vi "GetGpsData.vi"() -> (6 "latDeg":dbl format="%_6g", 7 "LonDeg":dbl format="%_6g", 8 "Sat":i32)   [LabVIEW 2017]
uses:
  <vilib>/Instr/_visa.llb/VISA Configure Serial Port (Instr).vi
  GlobalVarStop.vi
panel:
  out "Check":string
  out "error out":errorcluster
  out "Longitude (W)":dbl format="%#_8g"
  out "Latitude (N)":dbl format="%#_8g"
  out "Longitude [deg]":string
  out "Latitude [deg]":string
  in  "time zone":i32
  out "Time":string
  out "Mode":string
  out "Date [ddmmyy]":string
  out "Course over ground [degrees]":string
  out "Status":string
  out "Speed over ground [knots]":string
  out "E/W":string
  out "Longitude":string
  out "N/S":string
  out "Latitude":string
  out "UTC Time":string
  out "NMEA sentences":string
  # "GPS demo"
  # "[hhmmss.sss]"
  # "Floating Point Values"
  # "A = vAlid data\nV = inValid data"
  # "[ddmm.mmmm]"
  # "[dddmm.mmmm]"
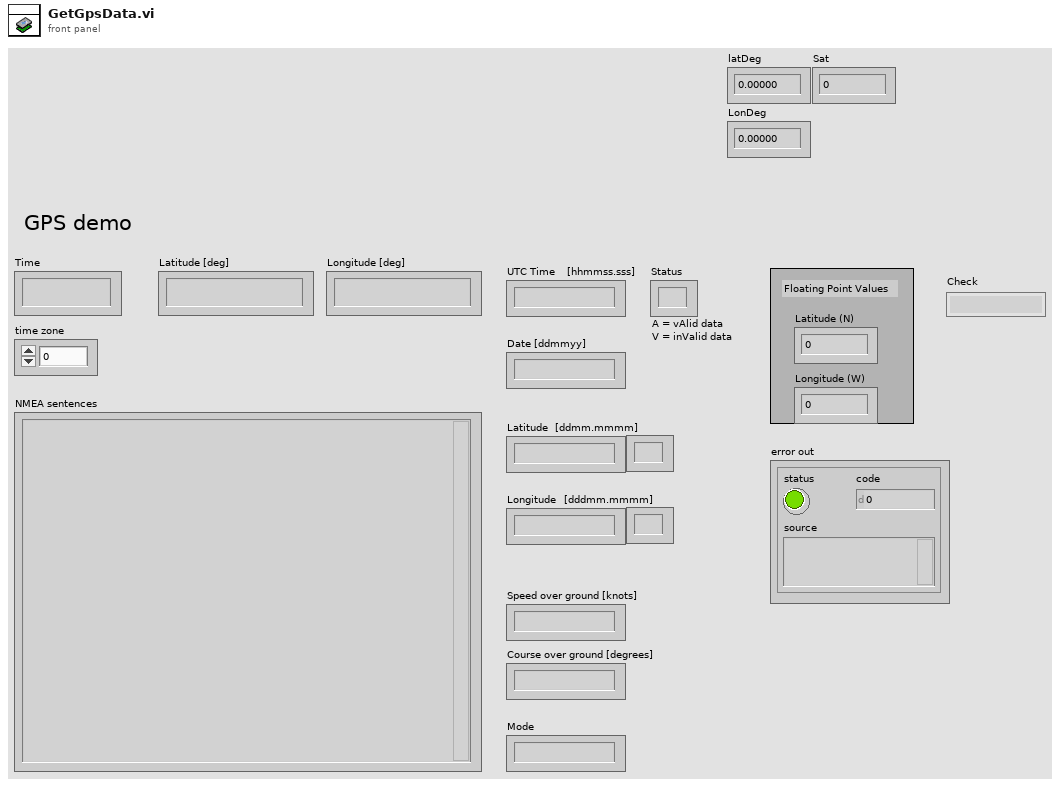
[diagram p1: front panel]
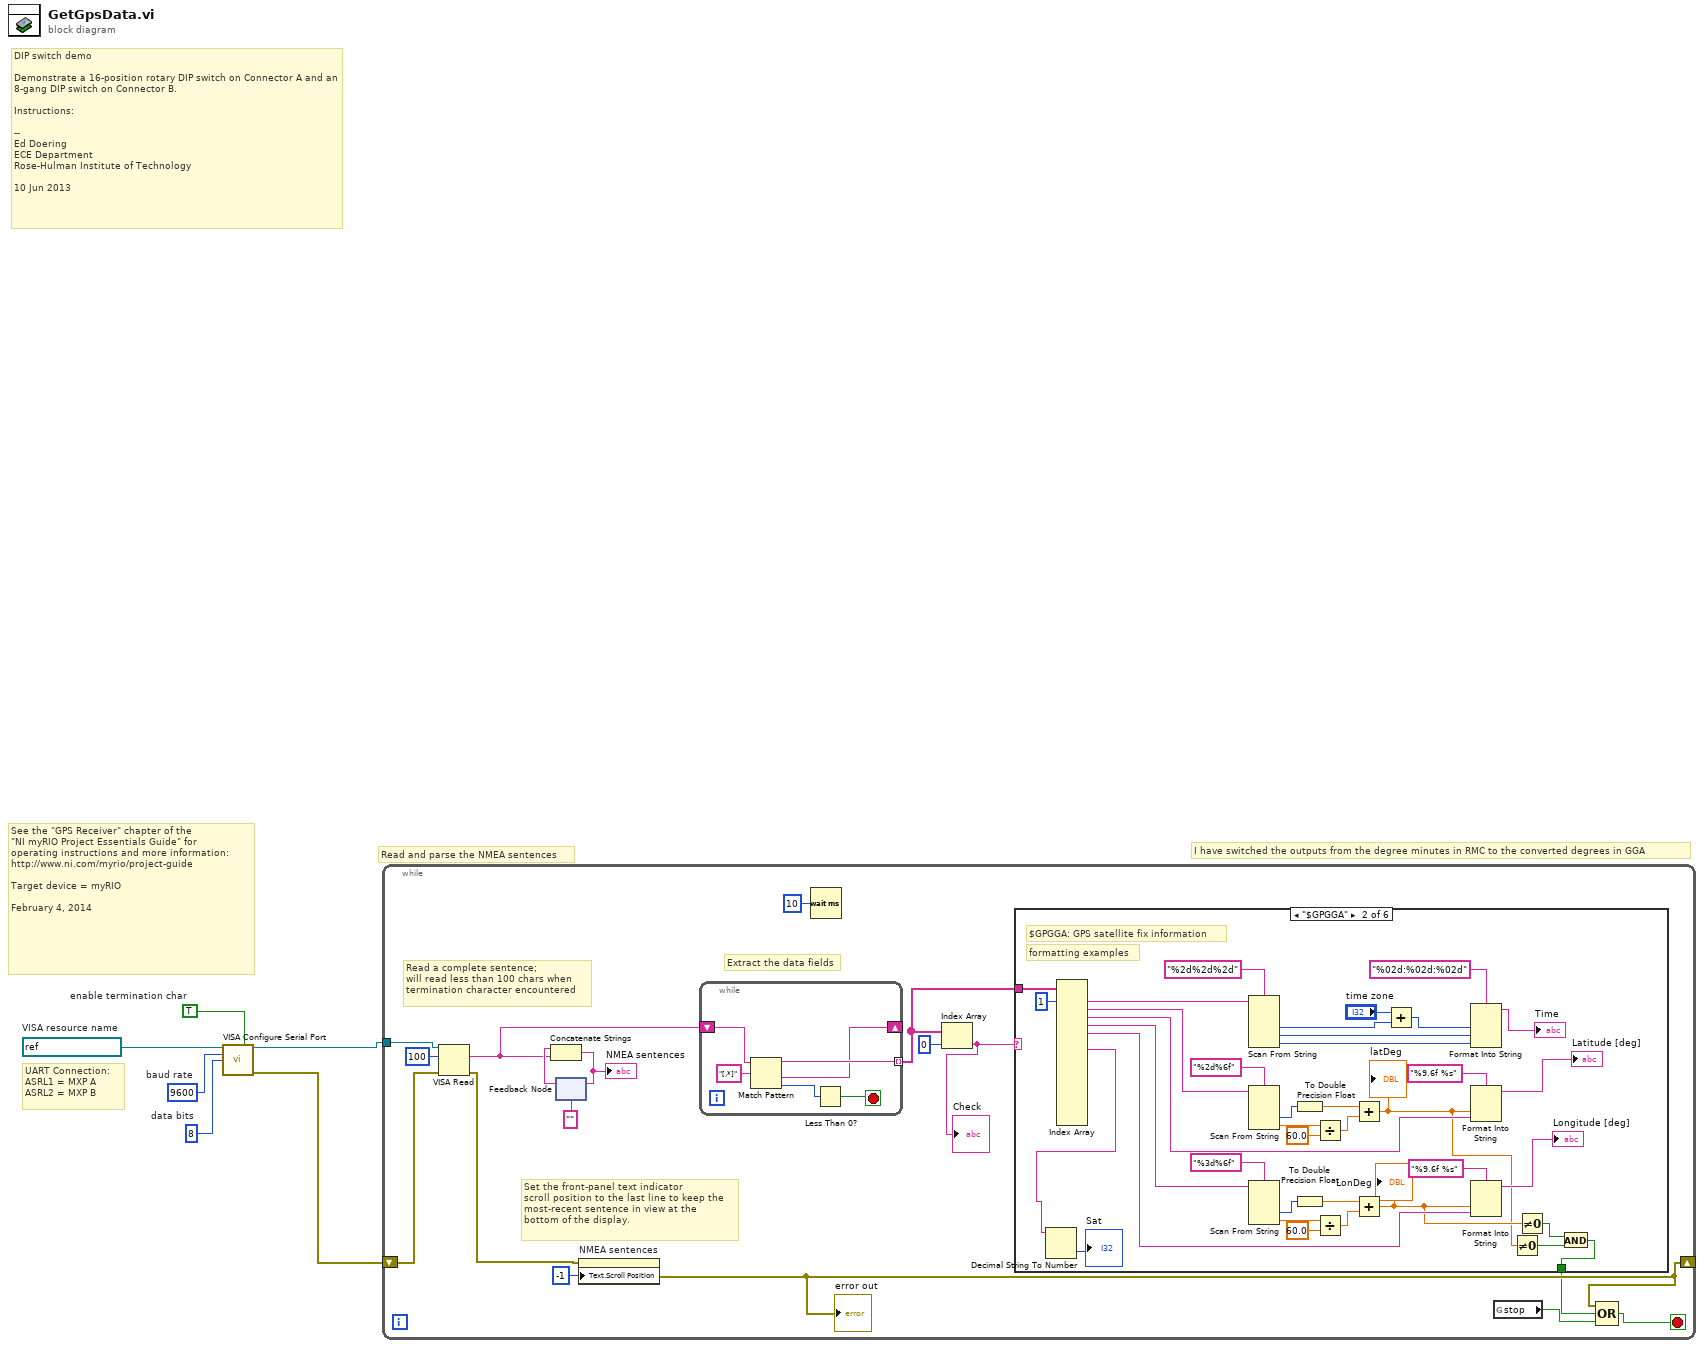
[diagram p0: block diagram]
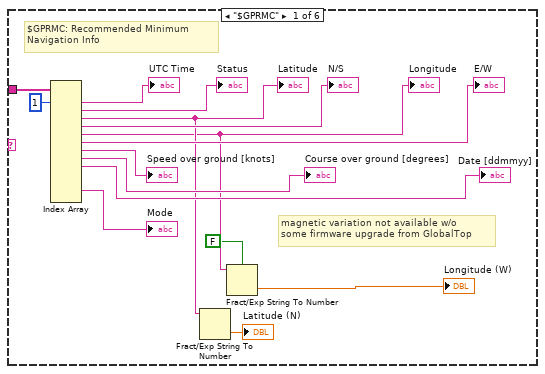
[diagram p2: hidden frame]
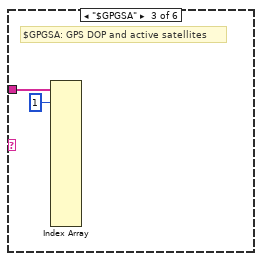
[diagram p3: hidden frame]
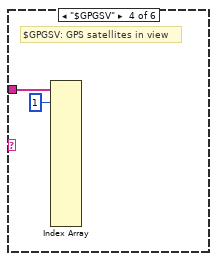
[diagram p4: hidden frame]
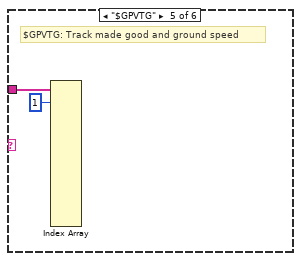
[diagram p5: hidden frame]
diagram:
  w2 = TRUE  # enable termination char
  w3 = u16 8  # data bits
  w4 = u32 9600  # baud rate
  w6 = refnum<visa-resource-name> "ASRL2::INSTR"  # VISA resource name
  # "I have switched the outputs from the degree minutes in RMC to the converted degrees in GGA"
  # "Read and parse the NMEA sentences"
  # "See the \"GPS Receiver\" chapter of the\n\"NI myRIO Project Essentials Guide\" for\noperating instructions and more information: \nhttp://www.ni.com/myrio/project-guide\n\nTarget device = myRIO\n\nFebruary 4, 2014"
  # "UART Connection:\nASRL1 = MXP A \nASRL2 = MXP B"
  # "DIP switch demo\n\nDemonstrate a 16-position rotary DIP switch on Connector A and an 8-gang DIP switch on Connector B.\n\nInstructions:\n\n-- \nEd Doering\nECE Department\nRose-Hulman Institute of Technology\n\n10 Jun 2013"
  n1 = call-poly "VISA Configure Serial Port"("VISA resource name"=w6, "Enable Termination\nChar (T)"=w2, "baud rate (9600)"=w4, "data bits (8)"=w3) -> ("VISA resource name out"=w5:refnum<visa-resource-name>, "error out"=w1:errorcluster)  [unwired: 10 in]
  n2 = while {
    tunnel: w5 -> [w23]
    shift-right: [w22] -> _
    shift-left: w1 -> [w21]
    stop <- w10 stop-if-true
    # "Set the front-panel text indicator\nscroll position to the last line to keep the\nmost-recent sentence in view at the\nbottom of the display."
    # "Extract the data fields"
    # "Read a complete sentence;\nwill read less than 100 chars when\ntermination character encountered"
    n3 = VISA Read(VISA resource name=w23, byte count=u32 100, error in (no error)=w21) -> (read buffer=w16:string, error out=w12:errorcluster)  [unwired: 2 out]
    n4 = feedback #1("") -> (w18:string)
    n5 = Concatenate Strings "Concatenate Strings"(w18, w16) -> (w20:string)
    "NMEA sentences" <- w20
    n6 = feedback-in #1(w20) -> ()
    n7 = property on="NMEA sentences" class="Str"(error in=w12, "Text.Scroll Position"=-1) -> (error out=w22:errorcluster)  [unwired: 1 in, 1 out]
    "error out" <- w22
    n8 = while {
      tunnel: [w86] -> w15 mode=indexing
      shift-right: [w85] -> _
      shift-left: w16 -> [w87]
      stop <- w84 stop-if-true
      n9 = Match Pattern(string=w87, regular expression="[,*]") -> (before substring=w86:string, after substring=w85:string, offset past match=w83:i32)  [unwired: 1 in, 1 out]
      n10 = Less Than 0?(x=w83) -> (x < 0?=w84:bool)
    }
    n11 = Wait (ms)(milliseconds to wait=u32 10) -> ()  [unwired: 1 out]
    n12 = Index Array "Index Array"(array=w15, index=0) -> (element=w7:string)
    "Check" <- w7
    n13 = case shown="\"$GPGGA\"" w7 {
      tunnel: w15 -> [w38 w76 w78 w80 w82 _]
      tunnel: [_ w41 _ _ _ _] -> w11
      frame "$GPRMC" {
        # "magnetic variation not available w/o\nsome firmware upgrade from GlobalTop"
        # "$GPRMC: Recommended Minimum\nNavigation Info"
        n14 = Index Array "Index Array"(array=w38, index #1=1 ("index")) -> (element #1=→"UTC Time":string, element #2=→"Status":string, element #3=w28:string, element #4=→"N/S":string, element #5=w27:string, element #6=→"E/W":string, element #7=→"Speed over ground [knots]":string, element #8=→"Course over ground [degrees]":string, element #9=→"Date [ddmmyy]":string, element #12=→"Mode":string)  [unwired: 12 in, 3 out]
        "Latitude" <- w28
        "Longitude" <- w27
        n15 = Fract/Exp String To Number(string=w28) -> (number=→"Latitude (N)":dbl)  [unwired: 3 in, 1 out]
        n16 = Fract/Exp String To Number(use system decimal point (T)=FALSE, string=w27) -> (number=→"Longitude (W)":dbl)  [unwired: 2 in, 1 out]
      }
      frame "$GPGGA" {
        # "formatting examples"
        # "$GPGGA: GPS satellite fix information"
        n17 = Index Array "Index Array"(array=w76, index #1=1 ("index")) -> (element #1=w73:string, element #2=w64:string, element #3=w57:string, element #4=w47:string, element #5=w46:string, element #7=w45:string)  [unwired: 15 in, 10 out]
        n18 = Decimal String To Number(string=w45) -> (number=→"Sat":i32)  [unwired: 2 in, 1 out]
        n19 = Scan From String "Scan From String"(format string="%2d%2d%2d", input string=w73) -> (output 1=w66:i32, output 2=w69:i32, output 3=w71:i32)  [unwired: 5 in, 3 out]
        n20 = Scan From String(format string="%2d%6f", input string=w64) -> (output 1=w61:i32, output 2=w63:dbl)  [unwired: 4 in, 3 out]
        n21 = Scan From String(format string="%3d%6f", input string=w47) -> (output 1=w51:i32, output 2=w49:dbl)  [unwired: 4 in, 3 out]
        n22 = To Double Precision Float(number=w61) -> (double precision float=w59:dbl)
        n23 = To Double Precision Float(number=w51) -> (double precision float=w53:dbl)
        n24 = Divide(x=w63, y=60.0) -> (x/y=w60:dbl)
        n25 = Divide(x=w49, y=60.0) -> (x/y=w52:dbl)
        n26 = Add(x=w59, y=w60) -> (x+y=w39:dbl)
        "latDeg" <- w39
        n27 = Add(x=w53, y=w52) -> (x+y=w40:dbl)
        "LonDeg" <- w40
        n28 = Add(x="time zone", y=w66) -> (x+y=w67:i32)
        n29 = Format Into String "Format Into String"(format string="%02d:%02d:%02d", w67, w69, w71) -> (resulting string=→"Time":string)  [unwired: 2 in, 1 out]
        n30 = Format Into String(format string="%9.6f %s", w39, w57) -> (resulting string=→"Latitude [deg]":string)  [unwired: 2 in, 1 out]
        n31 = Format Into String(format string="%9.6f %s", w40, w46) -> (resulting string=→"Longitude [deg]":string)  [unwired: 2 in, 1 out]
        n32 = Not Equal To 0?(x=w39) -> (x != 0?=w42:bool)
        n33 = Not Equal To 0?(x=w40) -> (x != 0?=w43:bool)
        n34 = And(x=w43, y=w42) -> (x .and. y?=w41:bool)
      }
      frame "$GPGSA" {
        # "$GPGSA: GPS DOP and active satellites"
        n35 = Index Array(array=w78, index #1=1 ("index")) -> ()  [unwired: 15 in, 16 out]
      }
      frame "$GPGSV" {
        # "$GPGSV: GPS satellites in view"
        n36 = Index Array(array=w80, index #1=1 ("index")) -> ()  [unwired: 15 in, 16 out]
      }
      frame "$GPVTG" {
        # "$GPVTG: Track made good and ground speed"
        n37 = Index Array(array=w82, index #1=1 ("index")) -> ()  [unwired: 15 in, 16 out]
      }
      frame Default {
      }
    }
    n38 = global read "GlobalVarStop.vi" "stop"() -> (w8:bool)
    n39 = Compound Arithmetic op=OR(w22, w11, w8) -> (w10:bool)
  }
